vi "arreglobidi1.vi"() -> ()   [LabVIEW 2011]
panel:
  out "Array 2":dbl[](array[numeric])
  out "SUMA DE COLUMNA":dbl
  in  "COLUMNA":dbl
  in  "LINEA":dbl
  out "SUMAlINEA":dbl
  out "Array":dbl[][](array[numeric])
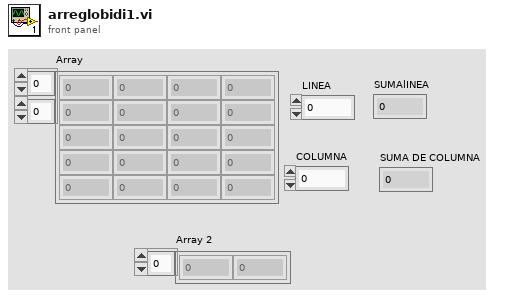
[diagram p1: front panel]
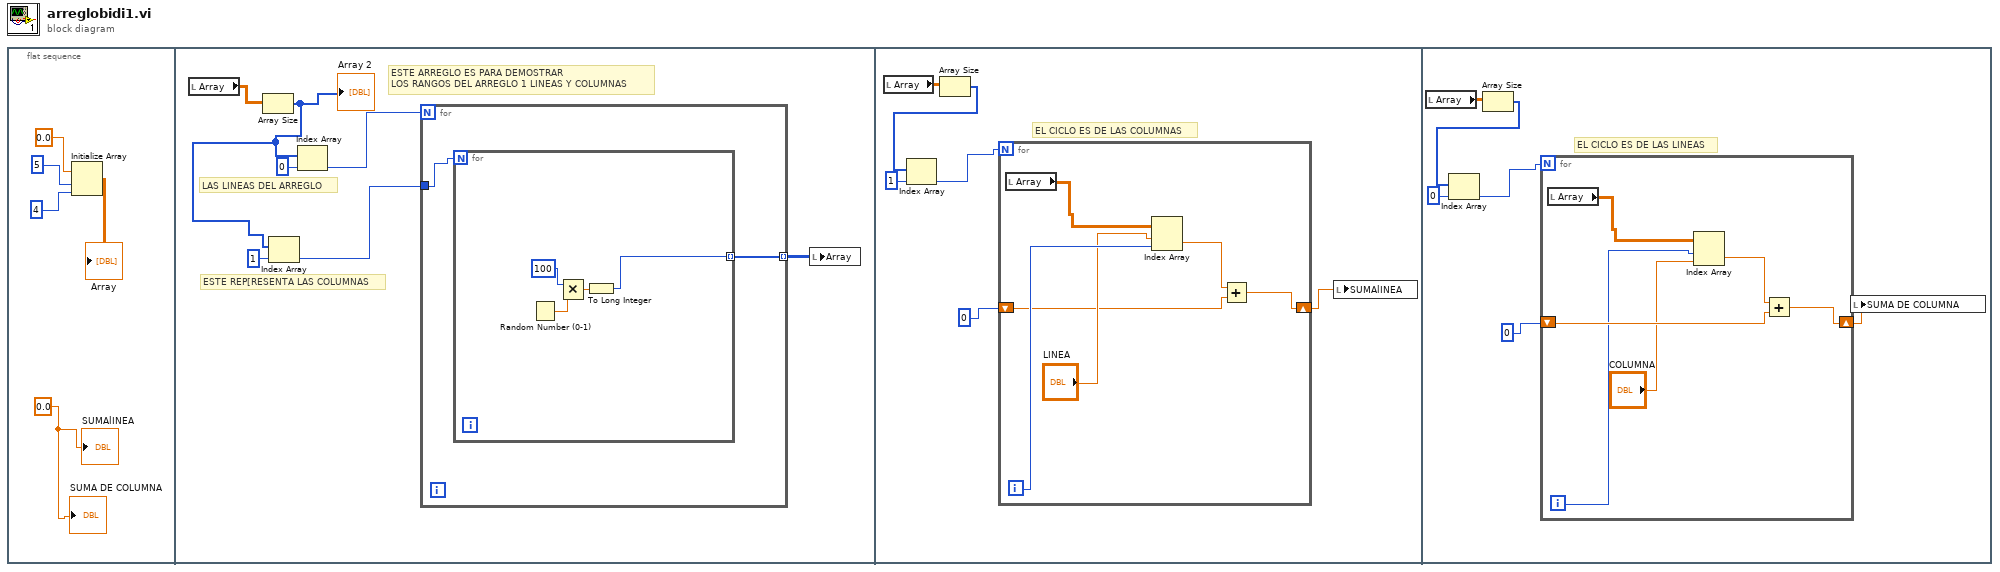
[diagram p0: block diagram]
diagram:
  n1 = flat-sequence {
    frame #0 {
      w1 = 0.0 ("element")
      n2 = Initialize Array "Initialize Array"(0.0 ("element"), 5 ("dimension size"), 4 ("dimension size")) -> (→"Array":dbl[][])
      "SUMAlINEA" <- w1
      "SUMA DE COLUMNA" <- w1
    }
    frame #1 {
      # "ESTE ARREGLO ES PARA DEMOSTRAR \nLOS RANGOS DEL ARREGLO 1 LINEAS Y COLUMNAS"
      # "ESTE REP[RESENTA LAS COLUMNAS"
      # "LAS LINEAS DEL ARREGLO"
      n3 = local read "Array"() -> (w11:dbl[][])
      n4 = Array Size(array=w11) -> (size(s)=w6:i32[])
      "Array 2" <- w6
      n5 = Index Array "Index Array"(array=w6, index=1) -> (element=w7:i32)
      n6 = Index Array "Index Array"(array=w6, index=0) -> (element=w8:i32)
      n7 = for {
        N: w8 -> [_]
        tunnel: [w14] -> w12 mode=indexing
        tunnel: w7 -> [w13]
        n8 = for {
          N: w13 -> [_]
          tunnel: [w15] -> w14 mode=indexing
          n9 = Random Number (0-1)() -> (number: 0 to 1=w18:dbl)
          n10 = Multiply(x=100, y=w18) -> (x*y=w16:dbl)
          n11 = To Long Integer(number=w16) -> (32bit integer=w15:i32)
        }
      }
      n12 = local write "Array"(w12) -> ()
    }
    frame #2 {
      # "EL CICLO ES DE LAS COLUMNAS"
      n13 = local read "Array"() -> (w24:dbl[][])
      n14 = Array Size(array=w24) -> (size(s)=w23:i32[])
      n15 = Index Array "Index Array"(array=w23, index=1) -> (element=w21:i32)
      n16 = for {
        N: w21 -> [_]
        shift-right: [w27] -> w19
        shift-left: 0 ("index") -> [w25]
        i -> [w29]
        n17 = local read "Array"() -> (w30:dbl[][])
        n18 = Index Array "Index Array"(array=w30, index (row)="LINEA", index (col)=w29) -> (element=w26:dbl)
        n19 = Add(x=w26, y=w25) -> (x+y=w27:dbl)
      }
      n20 = local write "SUMAlINEA"(w19) -> ()
    }
    frame #3 {
      # "EL CICLO ES DE LAS LINEAS"
      n21 = local read "Array"() -> (w31:dbl[][])
      n22 = Array Size(array=w31) -> (size(s)=w32:i32[])
      n23 = Index Array "Index Array"(array=w32, index=0) -> (element=w34:i32)
      n24 = for {
        N: w34 -> [_]
        shift-right: [w41] -> w36
        shift-left: 0 ("index") -> [w39]
        i -> [w38]
        n25 = local read "Array"() -> (w42:dbl[][])
        n26 = Index Array "Index Array"(array=w42, index (row)=w38, index (col)="COLUMNA") -> (element=w40:dbl)
        n27 = Add(x=w40, y=w39) -> (x+y=w41:dbl)
      }
      n28 = local write "SUMA DE COLUMNA"(w36) -> ()
    }
  }
